vi "CheckedShooter.vi"(5 "error in":errorcluster, 6 "Action":T4, 7 "Wait1":u32, 9 "Wait2":u32, 11 "Wait3":u32) -> (19 "error out":errorcluster)   [LabVIEW 2013]
doc: "CheckedShooter is used during a normal shooting sequence (either during one-ball autonomous or teleop). It controls the shooting pneumatics (through Shooter.vi), but it ALSO checks preconditions: the collector arm, the clappers, and the roller. It has the following actions:\n-Init: take two double solenoid references and store them (one for the clapper, one for the roller). Take two single solenoid references and use them to initialize Shooter.vi (one for the firing cylinder, one for the kicker).\n-Shoot:\n +Check if the collector is up (hitting the top limit switch). (Only if CheckLimitSwitch is true.)\n +Actuate the roller to out.\n +Actuate the clapper to middle.\n +Shoot (using Shooter.vi). Wait1, Wait2, and Wait3 correspond to the waits used by Shooter.vi."
uses:
  ShooterAction.ctl
  DoubleSolenoidControl.ctl
  CheckedShooterAction.ctl
  <vilib>/Rock Robotics/WPI/Solenoid/WPI_SolenoidChannel.ctl
  <vilib>/Rock Robotics/SystemInterfaces/Typedef/FPGA_TypedefSolenoidModule.ctl
  <vilib>/Rock Robotics/WPI/Solenoid/WPI_SolenoidDevRef.ctl
panel:
  in  "Roller":T1={"DevStatus"={"status"=FALSE, "code"=0, "source"=""}, "Solenoid Module"=enum."Solenoid Module 1", "Forward Solenoid Channel"=enum."Invalid", "Reverse Solenoid Channel"=enum."Invalid"}
  in  "Clapper":T1={"DevStatus"={"status"=FALSE, "code"=0, "source"=""}, "Solenoid Module"=enum."Solenoid Module 1", "Forward Solenoid Channel"=enum."Invalid", "Reverse Solenoid Channel"=enum."Invalid"}
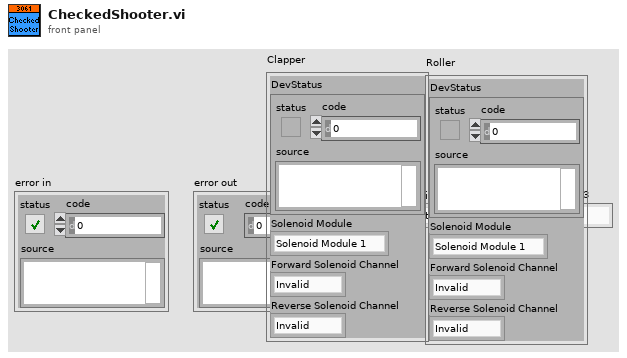
[diagram p1: front panel]
types:
  T1 = typedef "WPI_SolenoidDevRef.ctl" = cluster{"DevStatus":errorcluster, "Solenoid Module":T2, "Forward Solenoid Channel":T3, "Reverse Solenoid Channel":T3}
  T2 = typedef "FPGA_TypedefSolenoidModule.ctl" = enum16{"Solenoid Module 1", "Solenoid Module 2"}
  T3 = typedef "WPI_SolenoidChannel.ctl" = enum8{"Solenoid 1", "Solenoid 2", "Solenoid 3", "Solenoid 4", "Solenoid 5", "Solenoid 6", "Solenoid 7", "Solenoid 8", "Invalid"}
  T4 = typedef "CheckedShooterAction.ctl" = enum16{"Init", "Shoot"}
  T5 = typedef "DoubleSolenoidControl.ctl" = enum16{"Init", "Out", "In", "Middle"}
  T6 = typedef "ShooterAction.ctl" = enum16{"Init", "Shoot"}
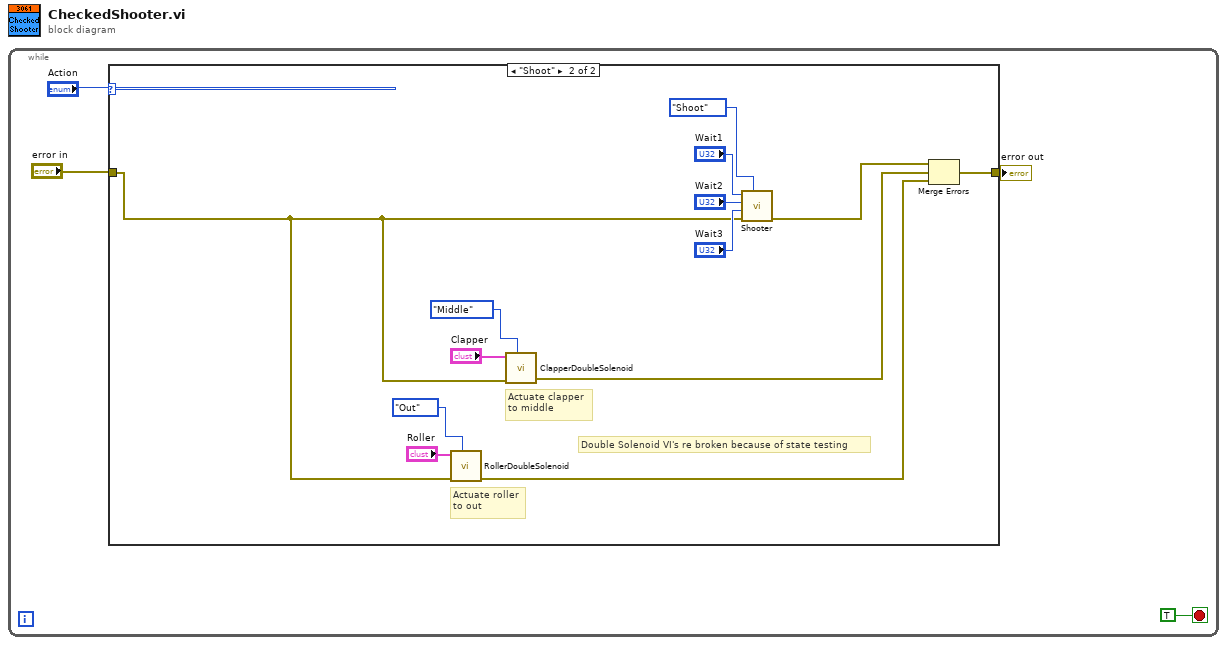
[diagram p0: block diagram]
diagram:
  n1 = while {
    stop <- TRUE stop-if-true
    n2 = case shown="\"Shoot\"" "Action" {
      tunnel: "error in" -> [w5 w10]
      tunnel: [w5 w7] -> w1
      frame "Init", Default {
      }
      frame "Shoot" {
        # "Double Solenoid VI's re broken because of state testing"
        # "Actuate clapper\nto middle"
        # "Actuate roller\nto out"
        n3 = call "RollerDoubleSolenoid.vi"("State"=DoubleSolenoidControl."Out", "Error in"=w10, "SolenoidDevRef"="Roller") -> ("Error out"=w8:errorcluster)  [unwired: 8 in]
        n4 = call "ClapperDoubleSolenoid.vi"("State"=DoubleSolenoidControl."Middle", "Error in"=w10, "SolenoidDevRef"="Clapper") -> ("Error out"=w9:errorcluster)  [unwired: 8 in]
        n5 = call "Shooter.vi"("Action"=ShooterAction."Shoot", "error in"=w10, "Wait3"="Wait3", "Wait2"="Wait2", "Wait1"="Wait1") -> ("error out"=w6:errorcluster)  [unwired: 6 in]
        n6 = Merge Errors(w6, w9, w8) -> (w7:errorcluster)
      }
    }
    "error out" <- w1
  }
